vi "ISEG_HVChannel.set Event Mask.vi"(0 "i ref in":refnum<vi>, 3 "Set EventMask":i32 format="%b", 5 "error in (no error)":errorcluster) -> (14 "i ref out":refnum<vi>, 19 "error out":errorcluster)   [LabVIEW 2014, in "ISEG_HVChannel.lvlib"]
doc: "This VI sets for all channels the event mask to 32 (fifth bit to 1) so that the board class can read the emergency_status."
uses:
  ISEG_HVChannel.lvlib
  CSCore/CSSystem/CoreLib/CoreLib.string 2 byte array.vi
  CSCore/CSSystem/CoreLib/CoreLib.int 2 byte array.vi
  CSCore/CSSystem/CoreLib/CoreLib.short 2 byte array.vi
  CSCore/CSApplicationBaseClasses/PSChannelBase/PSChannelBase.lvlib
  CSCore/CSSystem/CoreLib/CoreLib.lvlib
  CSCore/BaseProcess/BaseProcess.lvlib
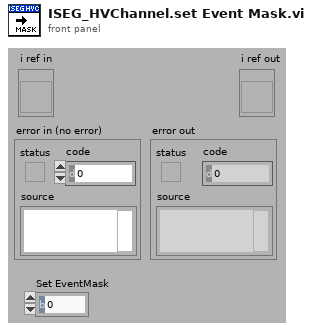
[diagram p1: front panel]
types:
  T1 = typedef "BaseProcess.lvlib/BaseProcess.i attribute.ctl" = cluster{"EventStatus":string, "EventError":i32, "PresetEvtWatchD":i32, "PresetPdcWatchD":i32, "EventTimeout":i32, "PeriodicInterval":i32, "Interface":string[], "Address":string[], "Special":string[], "PeriodicError":i32, "PeriodicStatus":string, "SuperProc":string, "Descriptors":T2[], "CaseRef":refnum<vi>, "PdcRef":refnum<vi>, "Thread Ref":refnum<vi>, "eventErrorID":i32, "eventStatusID":i32, "periodicErrorID":i32, "periodicStatusID":i32, "pdcCtrID":i32}
  T2 = typedef "BaseProcess.lvlib/BaseProcess.descriptor definition.ctl" = cluster{"selector":string, "descriptor":T3}
  T3 = typedef "BaseProcess.lvlib/BaseProcess.descriptor string definition.ctl" = string
  T4 = typedef "CoreDefs.rawDataType.ctl" = i8[]
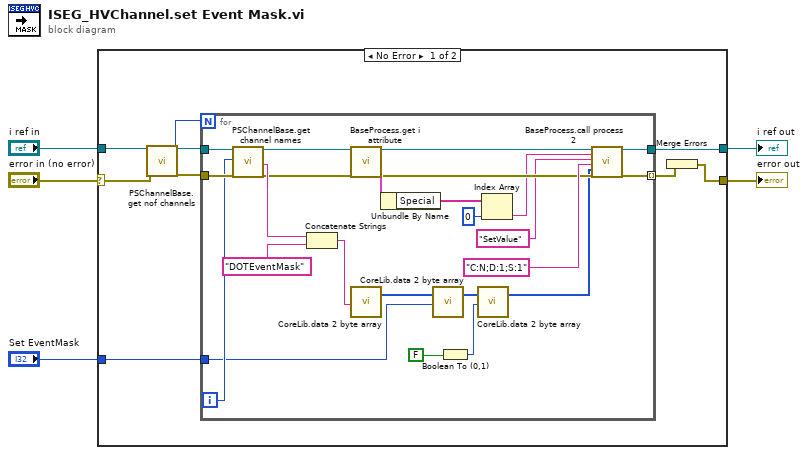
[diagram p0: block diagram]
diagram:
  n1 = case shown="No Error" "error in (no error)" {
    selector: "error in (no error)" -> [w11 w39]
    tunnel: "i ref in" -> [w7 w40]
    tunnel: "Set EventMask" -> [w14 _]
    tunnel: [w6 w40] -> w2
    tunnel: [w8 w39] -> w1
    frame No Error {
      n2 = call "PSChannelBase.get nof channels.vi"("i ref in"=w7, "error in (no error)"=w11) -> ("i ref out"=w13:refnum<vi>, "NofChannels"=w12:i32, "error out"=w10:errorcluster)  [unwired: 15 in]
      n3 = for {
        N: w12 -> [_]
        tunnel: w13 -> [w27]
        tunnel: w14 -> [w15]
        tunnel: w10 -> [w25]
        tunnel: [w21] -> w9 mode=indexing
        tunnel: [w19] -> w6
        i -> [w18]
        n4 = call "PSChannelBase.get channel names.vi"("i ref in"=w27, "channelIndex"=w18, "error in (no error)"=w25) -> ("i ref out"=w26:refnum<vi>, "logicalName"=w23:string, "error out"=w20:errorcluster)  [unwired: 13 in, 1 out]
        n5 = Concatenate Strings(w23, "DOTEventMask" ("string")) -> (w22:string)
        n6 = call "BaseProcess.get i attribute.vi"("i ref in"=w26, "error in (no error)"=w20) -> ("i ref out"=w34:refnum<vi>, "i attribute"=w36:T1, "error out"=w33:errorcluster)  [unwired: 15 in]
        n7 = call-poly "CoreLib.data 2 byte array.vi"("string"=w22) -> ("byteArray out"=w16:T4)  [unwired: 18 in]
        n8 = Unbundle By Name(w36) -> ("Special"=w38:string[])
        n9 = call-poly "CoreLib.data 2 byte array.vi"("byteArray"=w16, "i32"=w15) -> ("byteArray out"=w17:T4)  [unwired: 17 in]
        n10 = Boolean To (0,1)(Boolean=FALSE) -> (0, 1=w29:i16)
        n11 = call-poly "CoreLib.data 2 byte array.vi"("byteArray"=w17, "i16"=w29) -> ("byteArray out"=w28:T4)  [unwired: 17 in]
        n12 = Index Array(array=w38, index=0) -> (element=w32:string)
        n13 = call "BaseProcess.call process 2.vi"("i ref in"=w34, "Object"=w32, "Selector"="SetValue", "Data Descriptor"="C:N;D:1;S:1", "Data"=w28, "error in (no error)"=w33) -> ("i ref out"=w19:refnum<vi>, "error out"=w21:errorcluster)  [unwired: 12 in]
      }
      n14 = Merge Errors(w9) -> (w8:errorcluster)
    }
    frame Error {
    }
  }
  "error out" <- w1
  "i ref out" <- w2
